vi "Length_13.vi"() -> ()   [LabVIEW 2020]
uses:
  Support/Controls/Cmd_Mouse Popup.ctl
  Support/Controls/Clst_Initialize Input.ctl
  Support/Controls/Clst_Result inspec.ctl
  Support/Controls/Cmd_Var Data IO.ctl
  Variables/Global_Cal Info.vi
panel:
  out "Spec 2":string[][](table) caption="Spec (측정)"
  in  "Measured 3":string[][](table) caption="3. 원통도"
  out "직경":dbl caption="직경 (참고치)"
  out "볼지름":dbl caption="볼지름 (참고치)"
  out "기준 링 교정값":string
  in  "Measured 2":string[][](table) caption="1. 볼 지름 측정결과 (mm)"
  in  "명목값":string caption="교정 대상 명목값 (mm)"
  in  "기준 링 게이지":string(combo)="30 mm" caption="볼 지름 측정용 기준 링 게이지"
  out "기준기 분해능":string
  in  "Spec 변경":bool
  in  "Random":bool
  out "Spec":string[][](table) caption="Spec (명목 직경)"
  out "제목":string
  out "에러 출력":errorcluster
  out "Condition":string[][](table) caption="2. 직경 측정결과"
  in  "Measured":string[][](table) caption="지시편차 (μm)"
  out "Load?":bool
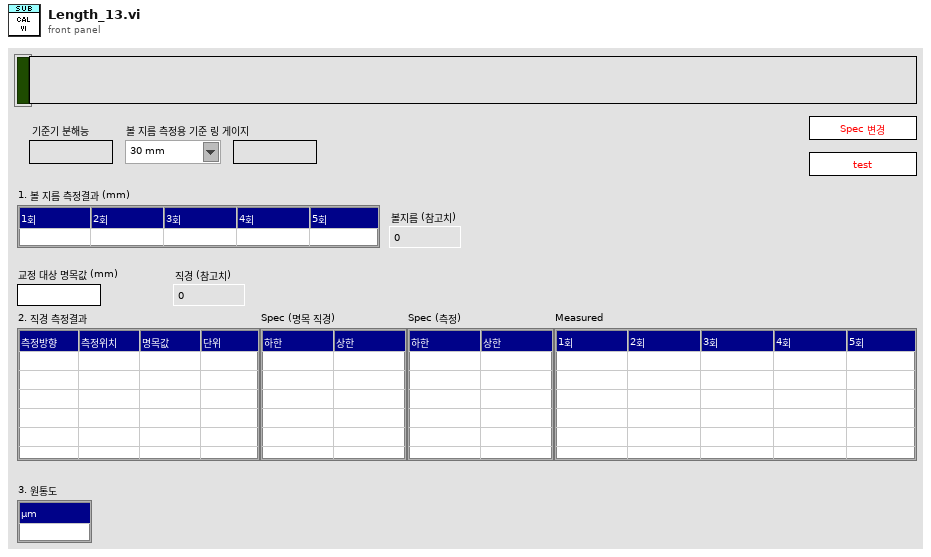
[diagram p1: front panel]
types:
  T1 = typedef "Cmd_Mouse Popup.ctl" = enum16{"활성화", "메뉴선택"}
  T2 = cluster{"Shift":bool, "Ctrl":bool, "Alt":bool, "Cmd":bool, "Opt":bool}
  T3 = typedef "Clst_Initialize Input.ctl" = cluster{"Initialize 1":cluster{"Condition":refnum<vi>[], "Spec":refnum<vi>[], "Measured":refnum<vi>[], "Resolution":refnum<vi>[], "Func_ext":string, "제목":refnum<vi>, "Measured_ADJ":refnum<vi>[]}, "Initialize 2":cluster{"문자열":refnum<vi>[], "콤보박스":refnum<vi>[], "링":refnum<vi>[], "열거형":refnum<vi>[], "테이블":refnum<vi>[], "여러열":refnum<vi>[], "디지털(DBL)":refnum<vi>[], "3D string":refnum<vi>[], "ctrl":refnum<vi>[], "boolean":refnum<vi>[]}}
  T4 = typedef "Clst_Result inspec.ctl" = cluster{"분해능":string, "문자열 1":string, "문자열 2":string, "숫자형 1":i32, "숫자형 2":i32, "숫자형 3":dbl, "문자배열 1D":string[], "문자배열 2D":string[][], "문자배열 3D":string[][][], "문자배열 4D":string[][][][], "불리언 1D":bool[]}
  T5 = typedef "Cmd_Var Data IO.ctl" = enum16{"Condition", "Condition Default", "Condition_Temp", "Resolution", "Resolution Default", "Resolution Old", "Spec", "Spec Default", "Spec Old", "Spec Temp", "Result", "Result2", "Result3", "Result_Temp", "Result_ADJ", "Result_ADJ2", "STD1", "STD2", "STD3", "STD4", "STD5", "STD Temp", "CMC", "CMC Default"}
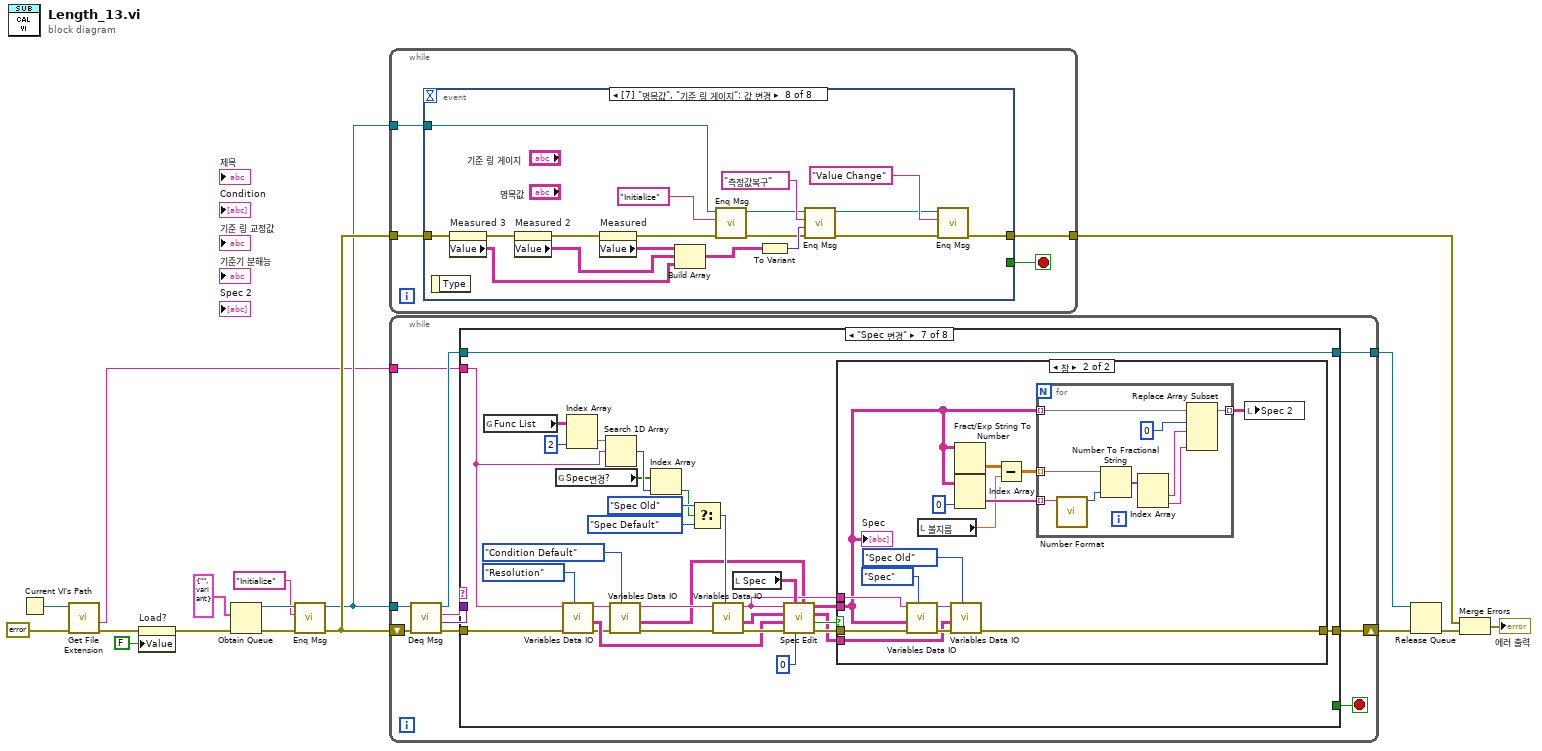
[diagram p0: block diagram]
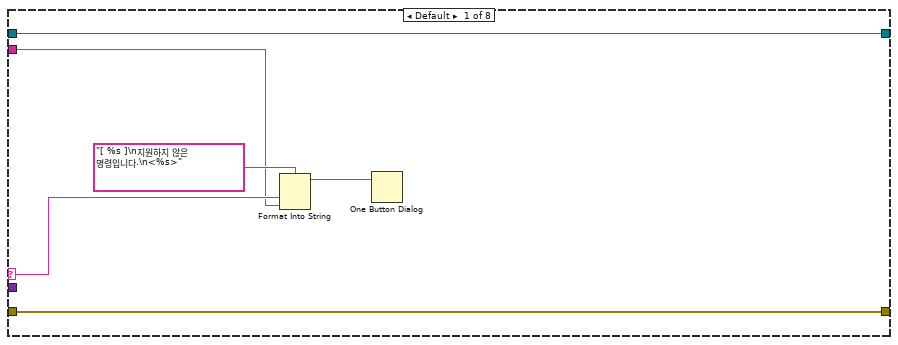
[diagram p2: hidden frame]
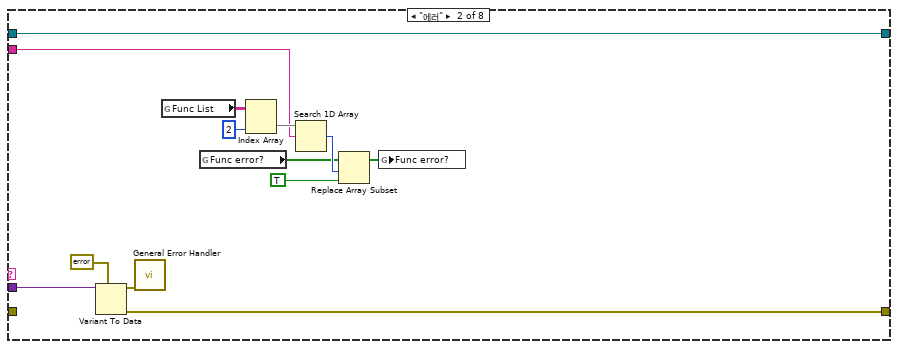
[diagram p3: hidden frame]
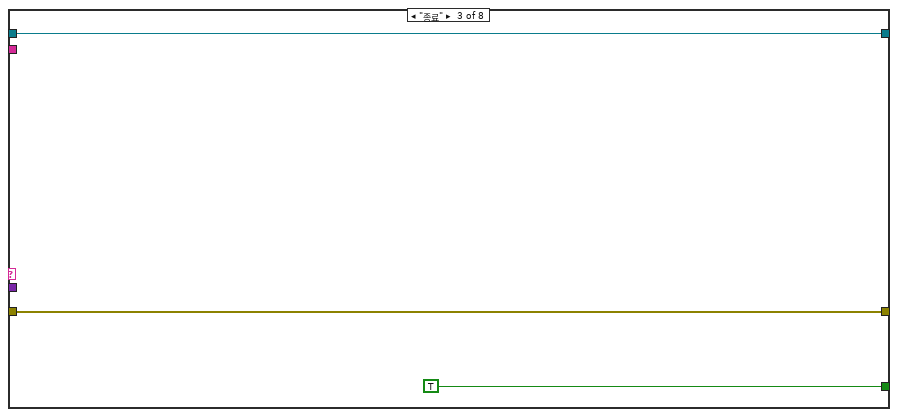
[diagram p4: hidden frame]
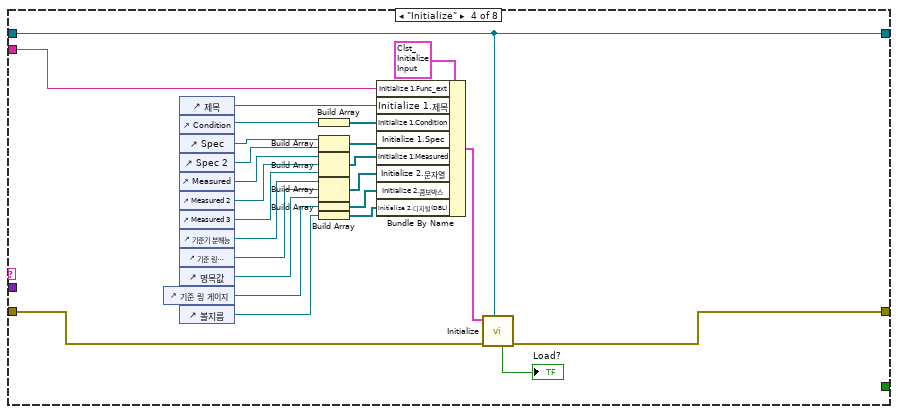
[diagram p5: hidden frame]
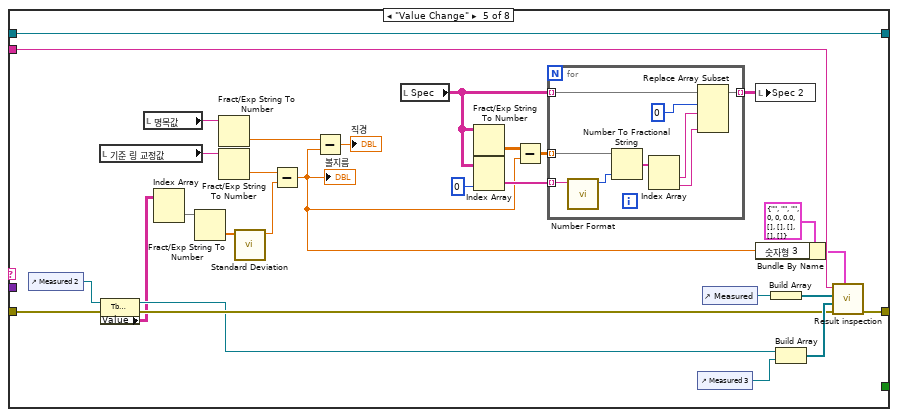
[diagram p6: hidden frame]
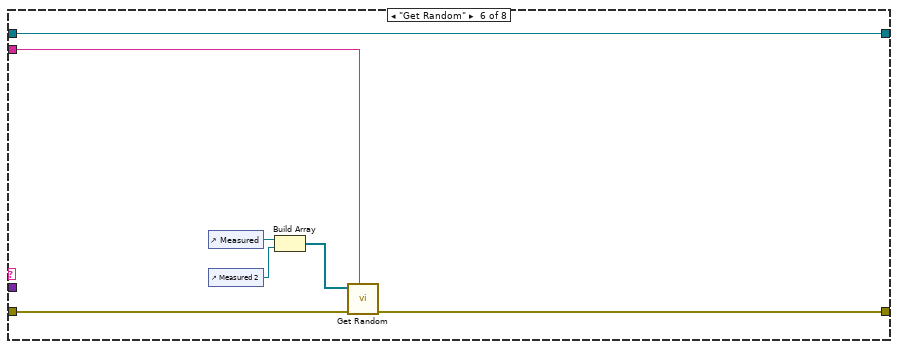
[diagram p7: hidden frame]
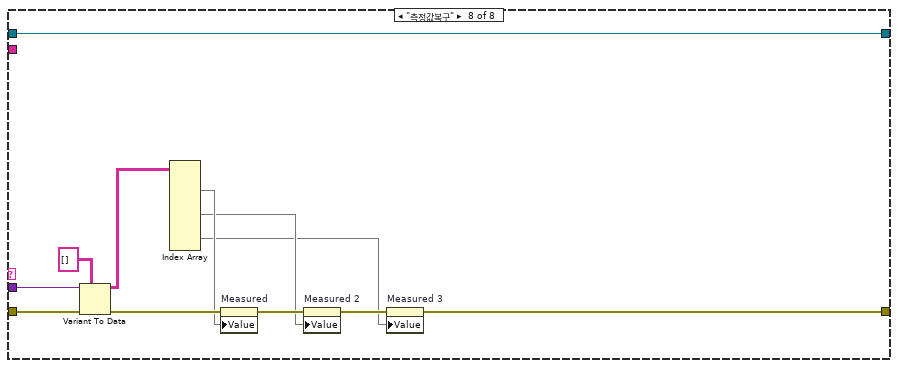
[diagram p9: hidden frame]
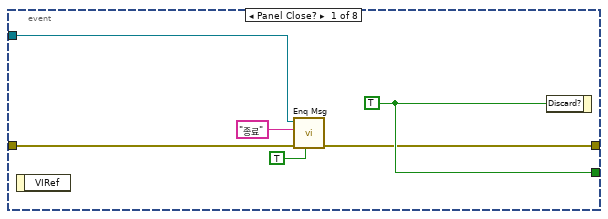
[diagram p10: hidden frame]
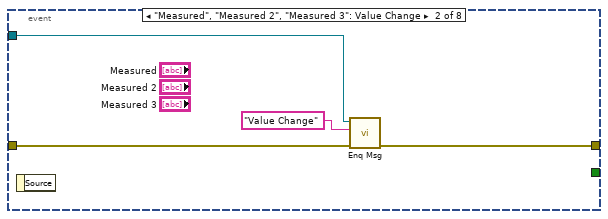
[diagram p11: hidden frame]
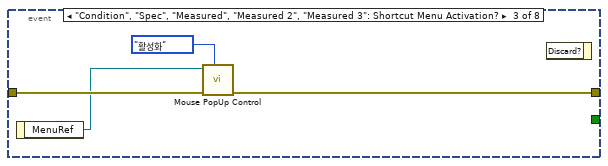
[diagram p12: hidden frame]
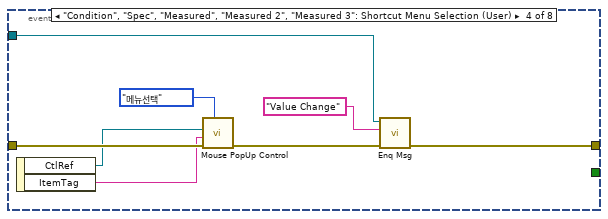
[diagram p13: hidden frame]
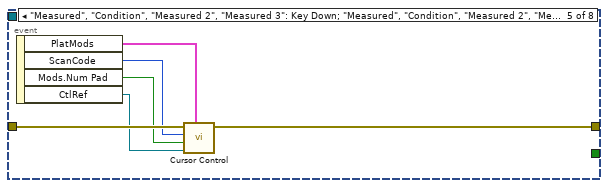
[diagram p14: hidden frame]
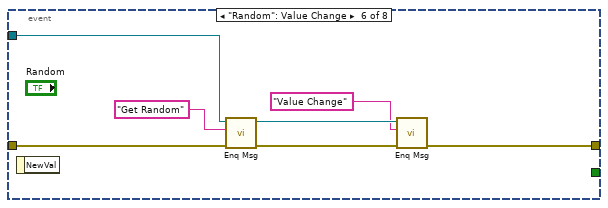
[diagram p15: hidden frame]
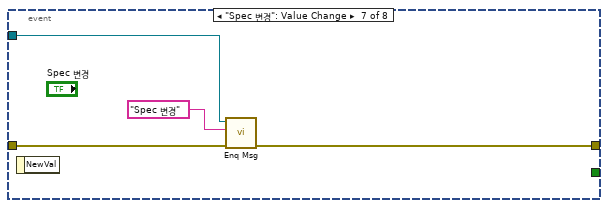
[diagram p16: hidden frame]
diagram:
  n1 = Current VI's Path() -> (path=w5:path)
  n2 = call <vilib>:"Get File Extension.vi"("error in (no error)"=errorcluster {"status"=FALSE, "code"=0, "source"=""} ("에러 상수"), "file"=w5) -> ("error out"=w3:errorcluster, "filename without extension"=w4:string)  [unwired: 5 in, 3 out]
  n3 = property on="Load?" class="Bool (엄격한)"(error in=w3, "Value"=FALSE ("Load?")) -> (error out=w2:errorcluster)  [unwired: 1 in, 1 out]
  n4 = Obtain Queue(element data type=cluster{"메세지":string, "값":variant} {"메세지"="", "값"=variant} ("Message Cluster"), error in (no error)=w2) -> (queue out=w14:refnum<queue>, error out=w16:errorcluster)  [unwired: 3 in, 1 out]
  n5 = call "Enq Msg.vi"("에러 입력(에러 없음)"=w16, "메세지"="Initialize", "큐 입력"=w14) -> ("에러 출력"=w15:errorcluster, "큐 출력"=w12:refnum<queue>)  [unwired: 7 in]
  n6 = while {
    tunnel: w15 -> [w19]
    tunnel: w12 -> [w20]
    tunnel: [w18] -> w9
    stop <- w21 stop-if-true
    n7 = event shown="[7] \"명목값\", \"기준 링 게이지\": 값 변경" {
      selector: _ -> [_ _ _ _ _ _ _ _]
      dyn-events: _ -> [_ _ _ _ _ _ _ _]
      timeout: _ -> [_ _ _ _ _ _ _ _]
      tunnel: [w27 _ _ _ _ _ _ _] -> w21
      tunnel: w20 -> [w25 w31 _ w36 _ w54 w58 w77]
      tunnel: w19 -> [w26 w29 w35 w43 w49 w55 w59 w67]
      tunnel: [w23 w30 w34 w37 w48 w50 w57 w61] -> w18
      event Panel Close? {
        w27 = TRUE ("버림?")
        n8 = event-data() -> ()  [unwired: 1 in, 1 out]
        n9 = call "Enq Msg.vi"("우선순위 메시지?"=TRUE, "에러 입력(에러 없음)"=w26, "메세지"="종료", "큐 입력"=w25) -> ("에러 출력"=w23:errorcluster)  [unwired: 6 in, 1 out]
        n10 = event-data("Discard?"=w27) -> ()  [unwired: 1 in, 1 out]
      }
      event "Measured", "Measured 2", "Measured 3": Value Change {
        n11 = event-data() -> ()  [unwired: 1 in, 1 out]
        n12 = call "Enq Msg.vi"("에러 입력(에러 없음)"=w29, "메세지"="Value Change", "큐 입력"=w31) -> ("에러 출력"=w30:errorcluster)  [unwired: 7 in, 1 out]
      }
      event "Condition", "Spec", "Measured", "Measured 2", "Measured 3": Shortcut Menu Activation? {
        n13 = event-data() -> ("MenuRef"=w33:refnum<k9>)  [unwired: 1 in]
        n14 = call "Mouse PopUp Control.vi"("type"=Cmd_Mouse_Popup."활성화", "error in"=w35, "메뉴 참조"=w33) -> ("error out"=w34:errorcluster)  [unwired: 8 in]
        n15 = event-data() -> ()  [unwired: 2 in, 1 out]
      }
      event "Condition", "Spec", "Measured", "Measured 2", "Measured 3": Shortcut Menu Selection (User) {
        n16 = event-data() -> ("CtlRef"=w41:refnum<vi>, "ItemTag"=w40:string)  [unwired: 1 in]
        n17 = call "Mouse PopUp Control.vi"("type"=Cmd_Mouse_Popup."메뉴선택", "error in"=w43, "아이템 태그"=w40, "Tbl 참조 번호"=w41) -> ("error out"=w38:errorcluster)  [unwired: 7 in]
        n18 = call "Enq Msg.vi"("에러 입력(에러 없음)"=w38, "메세지"="Value Change", "큐 입력"=w36) -> ("에러 출력"=w37:errorcluster)  [unwired: 7 in, 1 out]
      }
      event "Measured", "Condition", "Measured 2", "Measured 3": Key Down; "Measured", "Condition", "Measured 2", "Measured 3": Key Repeat {
        n19 = event-data() -> ("PlatMods"=w44:T2, "ScanCode"=w47:i16, "Mods.Num Pad"=w46:bool, "CtlRef"=w45:refnum<vi>)  [unwired: 1 in]
        n20 = call "Cursor Control.vi"("플랫폼 조합키"=w44, "참조"=w45, "Num Pad"=w46, "ScanCode"=w47, "error in"=w49) -> ("error out"=w48:errorcluster)  [unwired: 5 in, 1 out]
      }
      event "Random": Value Change {
        n21 = event-data() -> ()  [unwired: 1 in, 1 out]
        n22 = call "Enq Msg.vi"("에러 입력(에러 없음)"=w55, "메세지"="Get Random", "큐 입력"=w54) -> ("에러 출력"=w53:errorcluster, "큐 출력"=w52:refnum<queue>)  [unwired: 7 in]
        n23 = call "Enq Msg.vi"("에러 입력(에러 없음)"=w53, "메세지"="Value Change", "큐 입력"=w52) -> ("에러 출력"=w50:errorcluster)  [unwired: 7 in, 1 out]
      }
      event "Spec 변경": Value Change {
        n24 = event-data() -> ()  [unwired: 1 in, 1 out]
        n25 = call "Enq Msg.vi"("에러 입력(에러 없음)"=w59, "메세지"="Spec 변경", "큐 입력"=w58) -> ("에러 출력"=w57:errorcluster)  [unwired: 7 in, 1 out]
      }
      event "명목값", "기준 링 게이지": Value Change {
        n26 = event-data() -> ()  [unwired: 1 in, 1 out]
        n27 = property on="Measured 3" class="Tbl (엄격한)"(error in=w67) -> (error out=w66:errorcluster, "Value"=w65:string[][])  [unwired: 1 in, 1 out]
        n28 = property on="Measured 2" class="Tbl (엄격한)"(error in=w66) -> (error out=w76:errorcluster, "Value"=w69:string[][])  [unwired: 1 in, 1 out]
        n29 = property on="Measured" class="Tbl (엄격한)"(error in=w76) -> (error out=w75:errorcluster, "Value"=w70:string[][])  [unwired: 1 in, 1 out]
        n30 = Build Array(w70, w69, w65) -> (w68:string[][][])
        n31 = call "Enq Msg.vi"("에러 입력(에러 없음)"=w75, "메세지"="Initialize", "큐 입력"=w77) -> ("에러 출력"=w72:errorcluster, "큐 출력"=w71:refnum<queue>)  [unwired: 7 in]
        n32 = To Variant(anything=w68) -> (Variant=w74:variant)
        n33 = call "Enq Msg.vi"("에러 입력(에러 없음)"=w72, "값"=w74, "메세지"="측정값복구", "큐 입력"=w71) -> ("에러 출력"=w62:errorcluster, "큐 출력"=w63:refnum<queue>)  [unwired: 6 in]
        n34 = call "Enq Msg.vi"("에러 입력(에러 없음)"=w62, "메세지"="Value Change", "큐 입력"=w63) -> ("에러 출력"=w61:errorcluster)  [unwired: 7 in, 1 out]
      }
    }
  }
  n35 = while {
    shift-right: [w88] -> w11
    shift-left: w15 -> [w87]
    tunnel: w12 -> [w85]
    tunnel: [w80] -> w10
    tunnel: w4 -> [w79]
    stop <- w81 stop-if-true
    n36 = call "Deq Msg.vi"("에러 입력(에러 없음)"=w87, "큐 입력"=w85) -> ("에러 출력"=w86:errorcluster, "값"=w82:variant, "메세지"=w84:string, "큐 출력"=w83:refnum<queue>)  [unwired: 6 in]
    n37 = case shown="\"Spec 변경\"" w84 {
      selector: w84 -> [w90 _ _ _ _ _ _ _]
      tunnel: w86 -> [w94 _ w110 w135 w156 w176 w203 w244]
      tunnel: [w94 w104 w110 w127 w163 w177 w206 w237] -> w88
      tunnel: w83 -> [w93 w103 w108 w123 w164 w180 w210 w247]
      tunnel: w82 -> [_ w105 _ _ _ _ _ w245]
      tunnel: [_ _ TRUE ("버림?") _ _ _ _ _] -> w81
      tunnel: [w93 w103 w108 w123 w164 w180 w210 w247] -> w80
      tunnel: w79 -> [w89 w95 _ w124 w162 w175 w188 _]
      frame Default {
        n38 = Format Into String(format string="[ %s ]\n지원하지 않은 명령입니다.\n<%s>" ("메시지"), w90, w89) -> (resulting string=w91:string)  [unwired: 2 in, 1 out]
        n39 = One Button Dialog(message=w91) -> ()  [unwired: 1 in, 1 out]
      }
      frame "에러" {
        n40 = Variant To Data(type=errorcluster {"status"=FALSE, "code"=0, "source"=""} ("에러 출력"), Variant=w105) -> (data=w107:errorcluster, error out=w104:errorcluster)  [unwired: 1 in]
        n41 = call <vilib>:"General Error Handler.vi"("error in (no error)"=w107) -> ()  [unwired: 10 in, 5 out]
        n42 = global read "Global_Cal Info.vi" "Func List"() -> (w97:string[][])
        n43 = global read "Global_Cal Info.vi" "Func error?"() -> (w100:bool[])
        n44 = Index Array(array=w97, index (col)=2 ("비활성화된 인덱스 (열)")) -> (element=w98:string[])  [unwired: 1 in]
        n45 = Search 1D Array(1D array=w98, element=w95) -> (index of element=w101:i32)  [unwired: 1 in]
        n46 = Replace Array Subset(array=w100, new element=TRUE ("새 원소/부분배열"), index=w101) -> (w102:bool[])
        n47 = global write "Global_Cal Info.vi" "Func error?"(w102) -> ()
      }
      frame "종료" {
      }
      frame "Initialize" {
        n48 = control-ref of="기준 링 게이지"() -> (w120:refnum<vi>)
        n49 = control-ref of="제목"() -> (w128:refnum<vi>)
        n50 = control-ref of="Condition"() -> (w132:refnum<vi>)
        n51 = control-ref of="Spec"() -> (w126:refnum<vi>)
        n52 = control-ref of="Spec 2"() -> (w112:refnum<vi>)
        n53 = control-ref of="Measured"() -> (w129:refnum<vi>)
        n54 = control-ref of="Measured 2"() -> (w116:refnum<vi>)
        n55 = control-ref of="Measured 3"() -> (w115:refnum<vi>)
        n56 = control-ref of="기준기 분해능"() -> (w121:refnum<vi>)
        n57 = control-ref of="기준 링 교정값"() -> (w118:refnum<vi>)
        n58 = control-ref of="명목값"() -> (w117:refnum<vi>)
        n59 = control-ref of="볼지름"() -> (w114:refnum<vi>)
        n60 = Build Array(w132) -> (w131:refnum<vi>[])
        n61 = Build Array(w126, w112) -> (w125:refnum<vi>[])
        n62 = Build Array(w129, w116, w115) -> (w130:refnum<vi>[])
        n63 = Build Array(w121, w118, w117) -> (w122:refnum<vi>[])
        n64 = Build Array(w120) -> (w119:refnum<vi>[])
        n65 = Build Array(w114) -> (w113:refnum<vi>[])
        n66 = Bundle By Name(cluster=T3 {"Initialize 1"={"Condition"=[], "Spec"=[], "Measured"=[], "Resolution"=[], "Func_ext"="", "제목"=refnum, "Measured_ADJ"=[]}, "Initialize 2"={"문자열"=[], "콤보박스"=[], "링"=[], "열거형"=[], "테이블"=[], "여러열"=[], "디지털(DBL)"=[], "3D string"=[], "ctrl"=[], "boolean"=[]}} ("입력 클러스터"), "Initialize 1.Func_ext"=w124, "Initialize 1.제목"=w128, "Initialize 1.Condition"=w131, "Initialize 1.Spec"=w125, "Initialize 1.Measured"=w130, "Initialize 2.문자열"=w122, "Initialize 2.콤보박스"=w119, "Initialize 2.디지털(DBL)"=w113) -> (w133:T3)
        n67 = call "Initialize.vi"("큐 입력"=w123, "error in"=w135, "입력 클러스터"=w133) -> ("error out"=w127:errorcluster, "Load?"=→"Load?":bool)  [unwired: 5 in, 2 out]
      }
      frame "Value Change" {
        n68 = control-ref of="Measured 2"() -> (w154:refnum<vi>)
        n69 = local read "기준 링 교정값"() -> (w149:string)
        n70 = property class="Tbl (엄격한)"(reference=w154, error in=w156) -> (reference out=w153:refnum<vi>, error out=w155:errorcluster, "Value"=w152:string[][])
        n71 = local read "명목값"() -> (w146:string)
        n72 = Index Array(array=w152) -> (element=w151:string[])  [unwired: 2 in]
        n73 = Fract/Exp String To Number(string=w151) -> (number=w150:dbl[])  [unwired: 3 in, 1 out]
        n74 = Fract/Exp String To Number(string=w146) -> (number=w145:dbl)  [unwired: 3 in, 1 out]
        n75 = Fract/Exp String To Number(string=w149) -> (number=w148:dbl)  [unwired: 3 in, 1 out]
        n76 = call "Standard Deviation.vi"("X"=w150) -> ("mean"=w147:dbl)  [unwired: 8 in, 2 out]
        n77 = Subtract(x=w148, y=w147) -> (x-y=w137:dbl)
        "볼지름" <- w137
        n78 = Subtract(x=w145, y=w137) -> (x-y=→"직경":dbl)
        n79 = local read "Spec"() -> (w139:string[][])
        n80 = Fract/Exp String To Number(string=w139) -> (number=w142:dbl[][])  [unwired: 3 in, 1 out]
        n81 = Index Array(array=w139, index (col)=0 ("비활성화된 인덱스 (열)")) -> (element=w140:string[])  [unwired: 1 in]
        n82 = Subtract(x=w142, y=w137) -> (x-y=w141:dbl[][])
        n83 = for {
          tunnel: w139 -> [w173] mode=indexing
          tunnel: w141 -> [w171] mode=indexing
          tunnel: [w172] -> w136 mode=indexing
          tunnel: w140 -> [w166] mode=indexing
          n84 = call "Number Format.vi"("입력값"=w166) -> ("정밀도(단위적용)"=w165:i32)  [unwired: 10 in]
          n85 = Number To Fractional String(number=w171, precision (6)=w165) -> (F-format string=w170:string[])  [unwired: 2 in]
          n86 = Index Array(array=w170) -> (element #1=w169:string, element #2=w168:string)  [unwired: 2 in]
          n87 = Replace Array Subset(array=w173, new element #1=w169, index #1=0 ("인덱스"), new element #2=w168) -> (w172:string[])  [unwired: 1 in]
        }
        n88 = control-ref of="Measured 3"() -> (w143:refnum<vi>)
        n89 = control-ref of="Measured"() -> (w161:refnum<vi>)
        n90 = local write "Spec 2"(w136) -> ()
        n91 = Bundle By Name(cluster=T4 {"분해능"="", "문자열 1"="", "문자열 2"="", "숫자형 1"=0, "숫자형 2"=0, "숫자형 3"=0.0, "문자배열 1D"=[], "문자배열 2D"=[], "문자배열 3D"=[], "문자배열 4D"=[], "불리언 1D"=[]} ("입력 클러스터"), "숫자형 3"=w137) -> (w157:T4)
        n92 = Build Array(w161) -> (w160:refnum<vi>[])
        n93 = Build Array(w153, w143) -> (w159:refnum<vi>[])
        n94 = call "Result inspection.vi"("입력 클러스터"=w157, "error in"=w155, "Ref. Data (excluded)"=w159, "Ref. Data (Inspection)"=w160, "Func ext"=w162) -> ("error out"=w163:errorcluster)  [unwired: 3 in, 3 out]
      }
      frame "Get Random" {
        n95 = control-ref of="Measured"() -> (w179:refnum<vi>)
        n96 = control-ref of="Measured 2"() -> (w174:refnum<vi>)
        n97 = Build Array(w179, w174) -> (w178:refnum<vi>[])
        n98 = call "Get Random.vi"("Func_Ext"=w175, "에러 입력"=w176, "Meas"=w178) -> ("에러 출력"=w177:errorcluster)  [unwired: 7 in, 1 out]
      }
      frame "Spec 변경" {
        n99 = global read "Global_Cal Info.vi" "Func List"() -> (w193:string[][])
        n100 = global read "Global_Cal Info.vi" "Spec변경?"() -> (w189:bool[])
        n101 = call "Variables Data IO.vi"("Select"=Cmd_Var_Data_IO."Resolution", "error in"=w203, "Func_ext"=w188) -> ("error out"=w186:errorcluster, "Data Out"=w197:string[][], "Func_ext Out"=w184:string)  [unwired: 6 in]
        n102 = Index Array(array=w193, index (col)=2 ("비활성화된 인덱스 (열)")) -> (element=w191:string[])  [unwired: 1 in]
        n103 = Search 1D Array(1D array=w191, element=w188) -> (index of element=w190:i32)  [unwired: 1 in]
        n104 = call "Variables Data IO.vi"("Select"=Cmd_Var_Data_IO."Condition Default", "error in"=w186, "Func_ext"=w184) -> ("error out"=w185:errorcluster, "Data Out"=w181:string[][], "Func_ext Out"=w183:string)  [unwired: 6 in]
        n105 = Index Array(array=w189, index=w190) -> (element=w194:bool)
        n106 = Select(t=Cmd_Var_Data_IO."Spec Old" ("Select"), s=w194, f=Cmd_Var_Data_IO."Spec Default" ("Select")) -> (s? t:f=w187:T5)
        n107 = call "Variables Data IO.vi"("Select"=w187, "error in"=w185, "Func_ext"=w183) -> ("error out"=w205:errorcluster, "Data Out"=w198:string[][], "Func_ext Out"=w199:string)  [unwired: 6 in]
        n108 = local read "Spec"() -> (w200:string[][])
        n109 = call "Spec Edit.vi"("Condition"=w181, "열번호(기준값)"=0, "Spec Value"=w200, "에러 입력(에러 없음)"=w205, "Resolution"=w197, "Spec Default"=w198, "Func_ext"=w199) -> ("에러 출력"=w207:errorcluster, "변경?"=w208:bool, "Spec Default out"=w202:string[][], "Spec 출력"=w209:string[][])  [unwired: 1 in]
        n110 = case shown="참" w208 {
          tunnel: w209 -> [_ w213]
          tunnel: w207 -> [w211 w226]
          tunnel: [w211 w222] -> w206
          tunnel: w199 -> [_ w224]
          tunnel: w202 -> [_ w220]
          frame False {
          }
          frame True {
            n111 = call "Variables Data IO.vi"("Select"=Cmd_Var_Data_IO."Spec", "error in"=w226, "Data In"=w213, "Func_ext"=w224) -> ("error out"=w223:errorcluster, "Func_ext Out"=w221:string)  [unwired: 5 in, 1 out]
            n112 = local read "볼지름"() -> (w212:dbl)
            n113 = call "Variables Data IO.vi"("Select"=Cmd_Var_Data_IO."Spec Old", "error in"=w223, "Data In"=w220, "Func_ext"=w221) -> ("error out"=w222:errorcluster)  [unwired: 5 in, 2 out]
            n114 = Fract/Exp String To Number(string=w213) -> (number=w218:dbl[][])  [unwired: 3 in, 1 out]
            n115 = Index Array(array=w213, index (col)=0 ("비활성화된 인덱스 (열)")) -> (element=w216:string[])  [unwired: 1 in]
            n116 = Subtract(x=w218, y=w212) -> (x-y=w217:dbl[][])
            n117 = for {
              tunnel: w213 -> [w235] mode=indexing
              tunnel: w217 -> [w233] mode=indexing
              tunnel: [w234] -> w215 mode=indexing
              tunnel: w216 -> [w228] mode=indexing
              n118 = call "Number Format.vi"("입력값"=w228) -> ("정밀도(단위적용)"=w227:i32)  [unwired: 10 in]
              n119 = Number To Fractional String(number=w233, precision (6)=w227) -> (F-format string=w232:string[])  [unwired: 2 in]
              n120 = Index Array(array=w232) -> (element #1=w231:string, element #2=w230:string)  [unwired: 2 in]
              n121 = Replace Array Subset(array=w235, new element #1=w231, index #1=0 ("인덱스"), new element #2=w230) -> (w234:string[])  [unwired: 1 in]
            }
            n122 = local write "Spec 2"(w215) -> ()
            "Spec" <- w213
          }
        }
      }
      frame "측정값복구" {
        n123 = Variant To Data(error in=w244, type=string[][][] [], Variant=w245) -> (data=w242:string[][][], error out=w243:errorcluster)
        n124 = Index Array(array=w242) -> (element #1=w241:string[][], element #2=w239:string[][], element #3=w236:string[][])  [unwired: 9 in]
        n125 = property on="Measured" class="Tbl (엄격한)"(error in=w243, "Value"=w241) -> (error out=w240:errorcluster)  [unwired: 1 in, 1 out]
        n126 = property on="Measured 2" class="Tbl (엄격한)"(error in=w240, "Value"=w239) -> (error out=w238:errorcluster)  [unwired: 1 in, 1 out]
        n127 = property on="Measured 3" class="Tbl (엄격한)"(error in=w238, "Value"=w236) -> (error out=w237:errorcluster)  [unwired: 1 in, 1 out]
      }
    }
  }
  n128 = Release Queue(queue=w10, error in (no error)=w11) -> (error out=w8:errorcluster)  [unwired: 1 in, 2 out]
  n129 = Merge Errors(w9, w8) -> (→"에러 출력":errorcluster)
